vi "extract_gemini_embeddings.vi"(10 "body":string, 11 "headers":string) -> (0 "error out":errorcluster, 3 "vector response":refnum<class "message_vectors.lvclass">)   [LabVIEW 2020, in "llm_gemini_embedding.lvclass"]
uses:
  llm_gemini_embedding.lvclass
  message_vectors/message_vectors.lvclass
  message_vectors/embedding.ctl
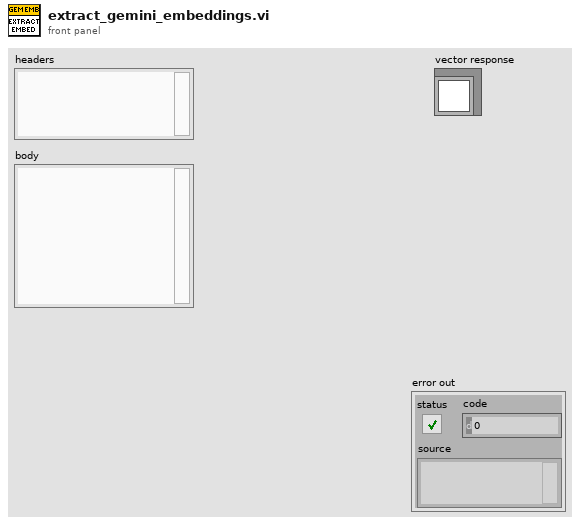
[diagram p1: front panel]
types:
  T1 = typedef "message_vectors.lvclass/embedding.ctl" = cluster{"index":u32, "Vectors":dbl[]}
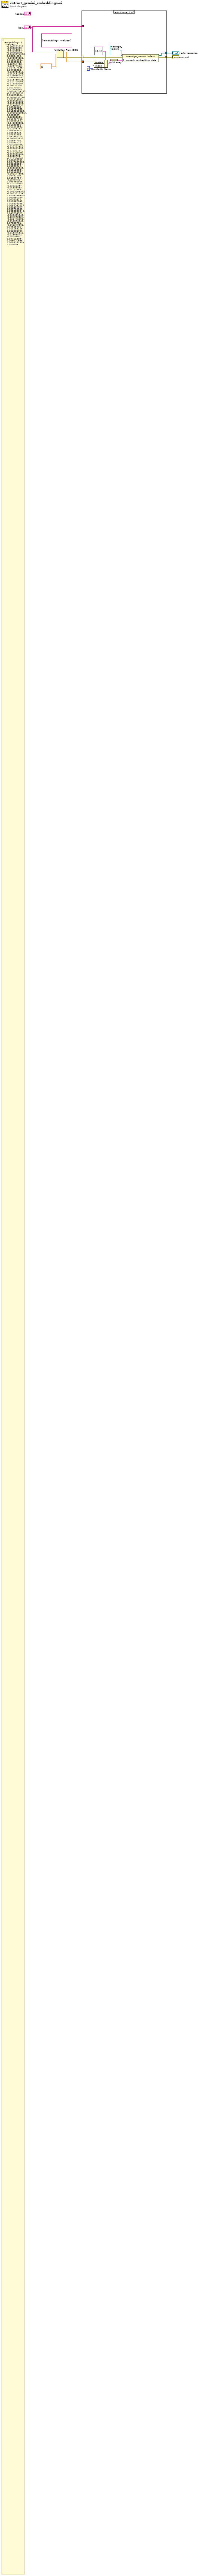
[diagram p0: block diagram]
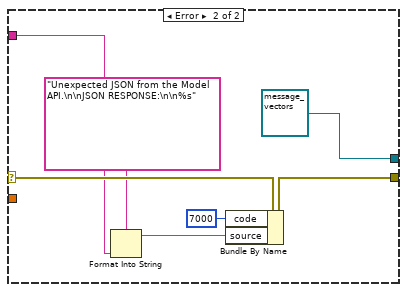
[diagram p2: hidden frame]
diagram:
  # "{\n  \"embedding\": {\n    \"values\": [\n      -0.047231518,\n      -0.08889983,\n      -0.04419314,\n      -0.06863804,\n      -0.0049074506,\n      0.03624099,\n      -0.009856856,\n      0.016243234,\n      0.04691866,\n      -0.03714493,\n      -0.03977612,\n      0.014977635,\n      0.04708513,\n      -0.035851516,\n      -0.062651105,\n      -0.033086166,\n      0.034998026,\n      -0.015499735,\n      -0.027729103,\n      -0.019559149,\n      -0.04751508,\n      0.01170116,\n      -0.02365999,\n      0.00016274797,\n      -0.019208992,\n      0.016236104,\n      -0.0014095766,\n      0.071379095,\n      -0.028982434,\n      -0.013108293,\n      -0.024488535,\n      0.08186968,\n      0.013737555,\n      0.0155369025,\n      -0.00091829314,\n      0.0088197,\n      -0.03925251,\n      0.016417766,\n      0.026036842,\n      -0.040938582,\n      0.016508564,\n      0.011262552,\n      -0.02148793,\n      0.004365512,\n      0.02315325,\n      0.07641439,\n      0.047487225,\n      -0.041815653,\n      0.023947027,\n      0.07093172,\n      0.029100286,\n      -0.013781425,\n      -0.029011693,\n      -0.07151152,\n      -0.012530245,\n      -0.025325404,\n      -0.0665756,\n      -0.010574568,\n      0.008093791,\n      0.0047687003,\n      0.001082584,\n      0.02356924,\n      -0.052512303,\n      0.013129984,\n      0.012122154,\n      -0.101144895,\n      0.04482109,\n      0.018477544,\n      -0.05454807,\n      0.053492308,\n      -0.027228562,\n      -0.03022357,\n      -0.06589853,\n      0.017729837,\n      -0.0059004985,\n      -0.0055510947,\n      1.9704248e-05,\n      0.009642188,\n      0.00781673,\n      0.010967842,\n      0.028939556,\n      0.0065565323,\n      0.052412827,\n      0.095790505,\n      0.0058880844,\n      0.043736327,\n      -0.009651348,\n      -0.084973834,\n      -0.021442696,\n      -0.010370368,\n      0.07838781,\n      -0.062349502,\n      0.045284014,\n      0.016188128,\n      0.062002707,\n      -0.015876511,\n      -0.02809542,\n      -0.0879802,\n      0.047113054,\n      0.009076988,\n      0.0045291334,\n      0.010004993,\n      -0.011340695,\n      -0.039352782,\n      0.044145793,\n      -0.040936094,\n      -0.00029900117,\n      -0.027124718,\n      0.012740982,\n      0.03218615,\n      0.0016550618,\n      -0.037553538,\n      0.06617439,\n      -0.00046049908,\n      0.00026397375,\n      -0.011919249,\n      0.021605562,\n      -0.0026010585,\n      -0.03269,\n      0.029753782,\n      -0.007946083,\n      -0.07442993,\n      -0.041761704,\n      0.043065194,\n      -0.00392033,\n      0.03346495,\n      0.0016607206,\n      -0.009605451,\n      -0.076612726,\n      0.003007562,\n      0.043999057,\n      -0.019927442,\n      0.02688831,\n      0.0020498498,\n      -0.03679367,\n      -0.030156627,\n      0.0256319,\n      -0.008001353,\n      0.03147421,\n      -0.010507646,\n      0.0107044475,\n      -0.041257225,\n      -0.05551192,\n      0.031317454,\n      -0.016617717,\n      -0.057018545,\n      -0.02573171,\n      0.011673803,\n      0.015998999,\n      0.032798614,\n      -0.0817594,\n      0.0073211812,\n      -0.029503807,\n      -0.03190019,\n      -0.021577513,\n      0.007041589,\n      0.11653872,\n      -0.0686841,\n      0.028716682,\n      -0.016977899,\n      0.0057007708,\n      -0.086078726,\n      0.0293652,\n      -0.007154061,\n      -0.06303945,\n      -0.05085766,\n      0.053365726,\n      -0.023274237,\n      -0.020364081,\n      -0.026675178,\n      -0.013142401,\n      -0.021234157,\n      0.03545736,\n      -0.04115562,\n      -0.02718835,\n      -0.018951379,\n      -0.028806148,\n      0.058838315,\n      -0.04117275,\n      -0.05802319,\n      0.046340227,\n      -0.0166392,\n      0.013014403,\n      0.02755629,\n      0.0156043125,\n      0.021419905,\n      0.0017869225,\n      -0.02660685,\n      0.011671384,\n      0.0102597745,\n      0.007660559,\n      -0.011449108,\n      0.03724493,\n      0.041772008,\n      0.0064039365,\n      -0.036601424,\n      -0.024244845,\n      0.035477515,\n      -0.00868271,\n      -0.025010014,\n      0.029916275,\n      0.017658193,\n      -0.03631049,\n      0.015306452,\n      -0.00842561,\n      -0.023675991,\n      -0.09458285,\n      -0.051404,\n      0.04596996,\n      0.008212901,\n      -0.030245822,\n      0.033935666,\n      -0.062577054,\n      -0.039110754,\n      0.015719201,\n      0.03755898,\n      0.06968693,\n      0.023477785,\n      -0.030339131,\n      -0.018753508,\n      -0.0003810906,\n      0.07227782,\n      0.07798196,\n      0.037254672,\n      -0.028025944,\n      0.043937728,\n      -0.00042884136,\n      0.019232411,\n      -0.008381093,\n      -0.03984897,\n      0.019230157,\n      0.003206017,\n      -0.0039937114,\n      -0.0033147277,\n      0.016422741,\n      -0.02040195,\n      0.037501033,\n      -0.01685987,\n      0.077160485,\n      0.031199312,\n      -0.007988469,\n      -0.035294157,\n      0.06656116,\n      -0.038195595,\n      0.054604635,\n      0.038943633,\n      0.028515097,\n      0.065668516,\n      -0.023878457,\n      -0.05423746,\n      -0.008632987,\n      -0.020460095,\n      -0.03517382,\n      0.041412592,\n      -0.049204376,\n      0.00026863467,\n      0.03431282,\n      -0.038991943,\n      0.014754657,\n      -0.035171214,\n      -0.067913026,\n      -0.07979969,\n      -0.03876082,\n      -0.065946884,\n      0.01579471,\n      -0.06905035,\n      0.024866443,\n      0.070994034,\n      0.06618148,\n      -0.038922835,\n      -0.0052705845,\n      -0.012318804,\n      0.014232801,\n      -0.044796187,\n      0.0143176345,\n      0.04572387,\n      0.011183113,\n      0.027771918,\n      -0.010320122,\n      -0.030205568,\n      0.025218181,\n      0.0040904665,\n      0.030510155,\n      -0.009915051,\n      0.012363607,\n      -0.03121901,\n      0.036895875,\n      -0.0011865405,\n      -0.0026070538,\n      -0.015205964,\n      0.0523498,\n      -0.00036048432,\n      0.047859427,\n      0.024802504,\n      0.033119943,\n      0.009768681,\n      -0.02626078,\n      0.020337146,\n      0.0358087,\n      0.025485726,\n      0.016763812,\n      0.06882429,\n      -0.07815283,\n      -0.0014488379,\n      -0.026506683,\n      -0.030965118,\n      -0.033194322,\n      -0.015235017,\n      -0.011729366,\n      -0.024582906,\n      0.0118237855,\n      0.02330175,\n      -0.022879062,\n      -0.041356575,\n      -0.018108407,\n      0.00417884,\n      -0.08078407,\n      -0.020710293,\n      -0.017763305,\n      -0.009073149,\n      0.015380309,\n      -0.030667324,\n      -0.034280077,\n      0.07408785,\n      0.007373002,\n      0.0038584745,\n      0.038436815,\n      -0.011360833,\n      0.049817983,\n      0.03592449,\n      0.010911892,\n      -0.032124683,\n      -0.0031659787,\n      -0.011615231,\n      0.009214718,\n      0.031285465,\n      -0.0038551716,\n      0.024097417,\n      0.079560675,\n      0.053466428,\n      0.017329723,\n      0.06044631,\n      0.039758462,\n      0.034157325,\n      -0.036050566,\n      -0.07265345,\n      0.0016312951,\n      0.018088553,\n      0.009442829,\n      -0.0036303997,\n      0.016639562,\n      -0.010166295,\n      0.031649977,\n      -0.0059157894,\n      -0.019426625,\n      -0.024669925,\n      -0.014009426,\n      0.03565991,\n      0.013587516,\n      0.008049275,\n      -0.031233922,\n      0.04168118,\n      0.008126483,\n      -0.013727842,\n      0.066327244,\n      -0.01448442,\n      -0.030835297,\n      0.058115244,\n      -0.04379792,\n      0.013308259,\n      -0.0053964593,\n      0.01845459,\n      -0.016267104,\n      0.049303193,\n      0.03020801,\n      -0.006580604,\n      0.0031130705,\n      0.0056053624,\n      0.0035709497,\n      -0.06369537,\n      0.020105686,\n      -0.051204376,\n      -0.0268727,\n      0.090644084,\n      0.06786626,\n      0.03807915,\n      -0.05808778,\n      -0.023865864,\n      0.009395917,\n      -0.0070471703,\n      -0.08144848,\n      0.03742919,\n      0.01380814,\n      -0.0031397855,\n      0.028667893,\n      0.004558673,\n      -0.062263016,\n      0.048522882,\n      0.02569847,\n      -0.008834046,\n      0.030596768,\n      0.0553526,\n      0.031929217,\n      -0.000889901,\n      -0.064015225,\n      -0.022818413,\n      0.01862191,\n      -0.029626768,\n      0.03405145,\n      -0.005217433,\n      -0.030788245,\n      0.012545984,\n      -0.052601907,\n      -0.011395909,\n      -0.060494367,\n      -0.024956185,\n      0.049884155,\n      -0.028972153,\n      -0.027555538,\n      -0.049305327,\n      0.0071484563,\n      -0.024679534,\n      -0.021282293,\n      -0.00955905,\n      -0.034028117,\n      -0.0460292,\n      -0.053379457,\n      0.019007383,\n      0.0027271502,\n      -0.058717612,\n      0.013740261,\n      -0.005614476,\n      -0.014060787,\n      0.011313937,\n      0.046617836,\n      0.029673222,\n      0.0069246073,\n      -0.05409941,\n      0.015170647,\n      -0.06598819,\n      -0.02479334,\n      -0.031063683,\n      0.018985521,\n      0.027025962,\n      -0.04205039,\n      0.010024586,\n      0.039863005,\n      -0.042389825,\n      0.028306365,\n      0.013394084,\n      -0.0009641853,\n      -0.072024055,\n      -0.0040330803,\n      0.018839994,\n      -0.050330035,\n      0.049958058,\n      -0.0003759181,\n      -0.011209632,\n      -0.028905684,\n      -0.030915417,\n      -0.06329864,\n      -0.014727671,\n      0.0729199,\n      -0.014336021,\n      0.0017632105,\n      -0.033897866,\n      -0.016556606,\n      0.03203619,\n      -0.0699831,\n      0.06886637,\n      0.029740307,\n      0.038759567,\n      0.0060110604,\n      -0.014662274,\n      -0.08479731,\n      0.03764743,\n      -0.0043692165,\n      0.06626694,\n      -0.027261255,\n      -0.023431815,\n      -0.0077913697,\n      0.009471104,\n      -0.056128647,\n      0.041448887,\n      0.069959715,\n      -0.054786157,\n      0.005910692,\n      -0.014865035,\n      0.010603641,\n      0.02536229,\n      0.012820763,\n      0.0009559305,\n      0.05439193,\n      -0.0370251,\n      0.050155606,\n      0.010728983,\n      -0.032833267,\n      0.021548824,\n      -0.030759579,\n      0.016099662,\n      0.060254455,\n      0.010268601,\n      -0.014552548,\n      -0.07243641,\n      -0.022966515,\n      -0.0060249073,\n      -0.027784634,\n      0.007574712,\n      0.004906042,\n      0.015892306,\n      0.026499694,\n      -0.0025695986,\n      -0.033768278,\n      -0.027476497,\n      0.006251158,\n      0.042277634,\n      -0.06288648,\n      0.017009022,\n      -0.008017085,\n      0.0032802876,\n      0.004246023,\n      -0.09129917,\n      -0.0026175994,\n      -0.03502188,\n      0.030079074,\n      -0.03602636,\n      -0.0029652668,\n      -0.032012872,\n      0.044116594,\n      0.0013970449,\n      -0.04920705,\n      0.07049836,\n      0.03832632,\n      0.041011147,\n      -0.0015273868,\n      0.04777171,\n      0.011860862,\n      -0.013378519,\n      0.00832525,\n      -0.0026463133,\n      0.058352623,\n      0.0061126496,\n      0.052226264,\n      -0.0049276045,\n      0.018276293,\n      -0.04237793,\n      -0.034193806,\n      0.038811136,\n      -0.03270767,\n      0.035315767,\n      0.0033701684,\n      -0.0016467057,\n      -0.01010759,\n      -0.041910026,\n      0.035234477,\n      -0.011230594,\n      -0.013029649,\n      -0.037077844,\n      -0.011848581,\n      0.013014367,\n      -0.012881313,\n      -0.034732472,\n      -0.019047204,\n      -0.027969362,\n      0.049003955,\n      0.013019209,\n      0.016312841,\n      0.09370749,\n      0.00742433,\n      -0.029010836,\n      0.034497097,\n      -0.010075377,\n      -0.00032687464,\n      -0.042222776,\n      0.022202885,\n      0.037821535,\n      -0.0081024,\n      0.021516595,\n      0.028619388,\n      -0.007584795,\n      -0.025255384,\n      0.03533629,\n      0.08029491,\n      -0.041689925,\n      -0.03979638,\n      -0.019300032,\n      0.0013459766,\n      -0.011130282,\n      0.0072221323,\n      -0.011403843,\n      0.036388256,\n      0.014784777,\n      0.019616082,\n      -0.028245913,\n      -0.004955207,\n      -0.02463564,\n      0.005481733,\n      0.0131259365,\n      0.039282404,\n      0.0037030273,\n      -0.014365021,\n      0.045976266,\n      0.022191968,\n      0.031907916,\n      -0.009986491,\n      -0.024059884,\n      -0.017438807,\n      -0.0140576465,\n      0.020262176,\n      -0.069490045,\n      0.009871845,\n      0.041493513,\n      0.037161052,\n      -0.035199877,\n      -0.041863244,\n      -0.0063131563,\n      -0.053904098,\n      0.009275199,\n      0.007196064,\n      0.026816148,\n      0.010052717,\n      0.04697123,\n      0.01824187,\n      0.050883997,\n      -0.105377436,\n      -0.030547747,\n      -0.04900724,\n      0.009819753,\n      -0.022150313,\n      -0.04527409,\n      -0.02579085,\n      -0.022517715,\n      -0.0041114087,\n      -0.01704833,\n      -0.013949187,\n      -0.0046888306,\n      0.018308429,\n      0.012571188,\n      -0.032964643,\n      0.026575085,\n      -0.039072543,\n      0.011645464,\n      0.04487075,\n      0.004304704,\n      -0.0020956134,\n      0.032845777,\n      0.023615025,\n      -0.03255095,\n      -0.004909702,\n      0.010795684,\n      0.04759185,\n      0.05171794,\n      -0.0031195125,\n      -0.020420626,\n      0.028029233,\n      -0.025378706,\n      -0.05375482,\n      0.037130345,\n      -0.011014371,\n      0.01287483,\n      -0.027875299,\n      -0.06491678,\n      0.048762094,\n      0.036389306,\n      0.015175325,\n      -0.018039672,\n      0.00016351495,\n      -0.03251298,\n      -0.016454205,\n      -0.039760448,\n      0.023280567,\n      -0.010497313,\n      0.0018647427,\n      0.044812452,\n      -0.025805656,\n      0.0053858594,\n      0.042781442,\n      -0.052853804,\n      -0.024076218,\n      0.018355018,\n      -0.018469596,\n      -0.049173802,\n      0.0050430875,\n      0.011513442,\n      0.0109477015,\n      -0.041519597,\n      0.07522517,\n      -0.07542197,\n      0.0040730746,\n      -0.0054917503,\n      0.03768143,\n      0.026879277,\n      -0.06926819,\n      0.03136373,\n      -0.035226654,\n      0.041424673,\n      -0.031337656,\n      0.06628029,\n      -0.014546587,\n      -0.021574693,\n      -0.0269143,\n      0.03744254,\n      -0.048587285,\n      0.004050264,\n      0.04356937,\n      -0.016140357,\n      -0.008725523,\n      0.0025264292,\n      -0.035638254,\n      -0.006105302,\n      0.016609436,\n      0.0048165135,\n      0.025783053,\n      0.044309158,\n      -0.00972398,\n      -0.0036724189,\n      -0.03622426,\n      0.03651635,\n      -0.0031606304,\n      0.01899843,\n      -0.025853105,\n      -0.028426068,\n      -0.00689019,\n      0.03173721,\n      -0.020176854,\n      0.059713557,\n      -0.014176791,\n      -0.015934022,\n      -0.028101137,\n      0.041806486,\n      0.026034823,\n      0.03140521,\n      0.008322731,\n      0.0006811402,\n      0.021644007,\n      0.014829937,\n      -0.059517983,\n      0.006123095,\n      0.00090790837,\n      -0.00013320986,\n      0.013579158,\n      0.029412268,\n      -0.019696236,\n      -0.034617677,\n      -0.005011575,\n      0.04056732,\n      -0.050779726,\n      -0.054239813,\n      -0.012819067,\n      -0.023833515,\n      -0.014071193,\n      0.013370282,\n      0.034834445,\n      -0.007731518,\n      0.06514479,\n      -0.029679086,\n      0.056208774,\n      -0.008614089,\n      0.0050697145,\n      -0.029357282,\n      -0.03981249,\n      0.08600809,\n      -0.02215354,\n      0.10355234,\n      -0.027933871,\n      0.049165912,\n      -0.036430743,\n      0.06479266\n    ]\n  }\n}"
  n1 = Unflatten From JSON(path=string[] ["embedding", "values"], JSON string="body", type and defaults=dbl[] []) -> (value=w5:dbl[], error out=w2:errorcluster)  [unwired: 4 in]
  n2 = case shown="No Error" w2 {
    selector: w2 -> [w11 w22]
    tunnel: w5 -> [w14 _]
    tunnel: [w10 refnum<class "message_vectors.lvclass"> refnum ("message_vectors.lvclass")] -> w4
    tunnel: [w9 w17] -> w3
    tunnel: "body" -> [_ w21]
    frame No Error {
      n3 = Bundle By Name(cluster=T1 {"index"=0, "Vectors"=[]} ("embedding"), "Vectors"=w14, "index"=u32 0) -> (w13:T1)
      n4 = Build Array(w13) -> (w12:T1[])
      n5 = property class="message_vectors.lvclass"(reference=refnum<class "message_vectors.lvclass"> refnum ("message_vectors.lvclass"), error in=w11, "property:embedding_data"=w12) -> (reference out=w10:refnum<class "message_vectors.lvclass">, error out=w9:errorcluster)
    }
    frame Error {
      n6 = Format Into String(format string="Unexpected JSON from the Model API.\n\nJSON RESPONSE:\n\n%s", w21) -> (resulting string=w19:string)  [unwired: 2 in, 1 out]
      n7 = Bundle By Name(cluster=w22, "code"=7000, "source"=w19) -> (w17:errorcluster)
    }
  }
  "vector response" <- w4
  "error out" <- w3
